vi "Initialize Drive System.vi"(6 "RightDriveMaster":u8, 7 "LeftDriveMaster":u8, 8 "RightDriveSlave1":u8, 9 "RightDriveSlave2":u8, 10 "LeftDriveSlave 2":u8, 11 "LeftDriveSlave1":u8) -> (1 "RightDriveMaster":T1, 2 "LeftDriveMaster":T1)   [LabVIEW 2018]
uses:
  <vilib>/Rock Robotics/WPI/MotorControl/WPI_MotorControlDeviceRef.ctl
  <vilib>/Rock Robotics/WPI/MotorControl/WPI_MotorControlType.ctl
  <vilib>/Rock Robotics/SystemInterfaces/DIO/FPGA_DIOPWMChannel.ctl
  <vilib>/Rock Robotics/WPI/PWM/WPI_PWMDeadband.ctl
  <vilib>/Rock Robotics/SystemInterfaces/DIO/FPGA_DIOChannel.ctl
  <vilib>/Rock Robotics/WPI/ThirdParty/Phoenix-LabVIEW/Motor Controller/Controls/CTRE_Phoenix_MotorControl_NeutralMode.ctl
  Infrastructure/Constants.vi
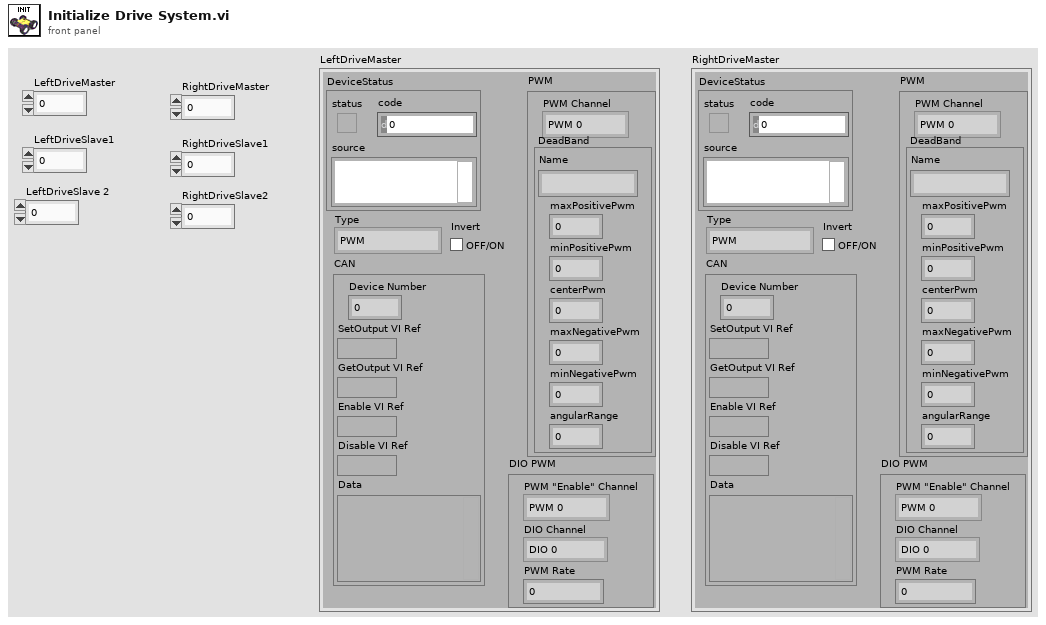
[diagram p1: front panel]
types:
  T1 = typedef "WPI_MotorControlDeviceRef.ctl" = cluster{"DeviceStatus":errorcluster, "Type":T2, "PWM":cluster{"PWM Channel":T3, "DeadBand":T4}, "CAN":cluster{"Device Number":u8, "SetOutput VI Ref":variant, "GetOutput VI Ref":variant, "Enable VI Ref":variant, "Disable VI Ref":variant, "Data":variant}, "Invert":bool, "DIO PWM":cluster{"PWM \"Enable\" Channel":T3, "DIOChannel":T5, "PWM Rate":dbl}}
  T2 = typedef "WPI_MotorControlType.ctl" = enum16{"PWM", "CAN", "DIO PWM"}
  T3 = typedef "FPGA_DIOPWMChannel.ctl" = enum8{"PWM 0", "PWM 1", "PWM 2", "PWM 3", "PWM 4", "PWM 5", "PWM 6", "PWM 7", "PWM 8", "PWM 9", "PWM MXP 0", "PWM MXP 1", "PWM MXP 2", "PWM MXP 3", "PWM MXP 4", "PWM MXP 5", "PWM MXP 6", "PWM MXP 7", "PWM MXP 8", "PWM MXP 9", "Invalid"}
  T4 = typedef "WPI_PWMDeadband.ctl" = cluster{"Name":string, "maxPositivePwm":i32, "minPositivePwm":i32, "centerPwm":i32, "maxNegativePwm":i32, "minNegativePwm":i32, "angularRange":u16}
  T5 = typedef "FPGA_DIOChannel.ctl" = enum8{"DIO 0", "DIO 1", "DIO 2", "DIO 3", "DIO 4", "DIO 5", "DIO 6", "DIO 7", "DIO 8", "DIO 9", "DIO MXP 0", "DIO MXP 1", "DIO MXP 2", "DIO MXP 3", "DIO MXP 4", "DIO MXP 5", "DIO MXP 6", "DIO MXP 7", "DIO MXP 8", "DIO MXP 9", "DIO MXP 10", "DIO MXP 11", "DIO MXP 12", "DIO MXP 13", "DIO MXP 14", "DIO MXP 15", "SPI Port CS1", "SPI Port CS2", "SPI Port CS3", "SPI Port MISO", "SPI Port MOSI", "Invalid"}
  T6 = typedef "CTRE_Phoenix_MotorControl_NeutralMode.ctl" = enum8{"EEPROMSetting", "Override to Coast", "Override to Brake"}
  T7 = enum16{"FollowerType_PercentOutput", "FollowerType_AuxOutput1"}
  T8 = cluster{"Cruise Velocity":i32, "Acceleration":i32}
  T9 = cluster{"P":dbl, "I":dbl, "D":dbl, "F":dbl, "I Zone":dbl}
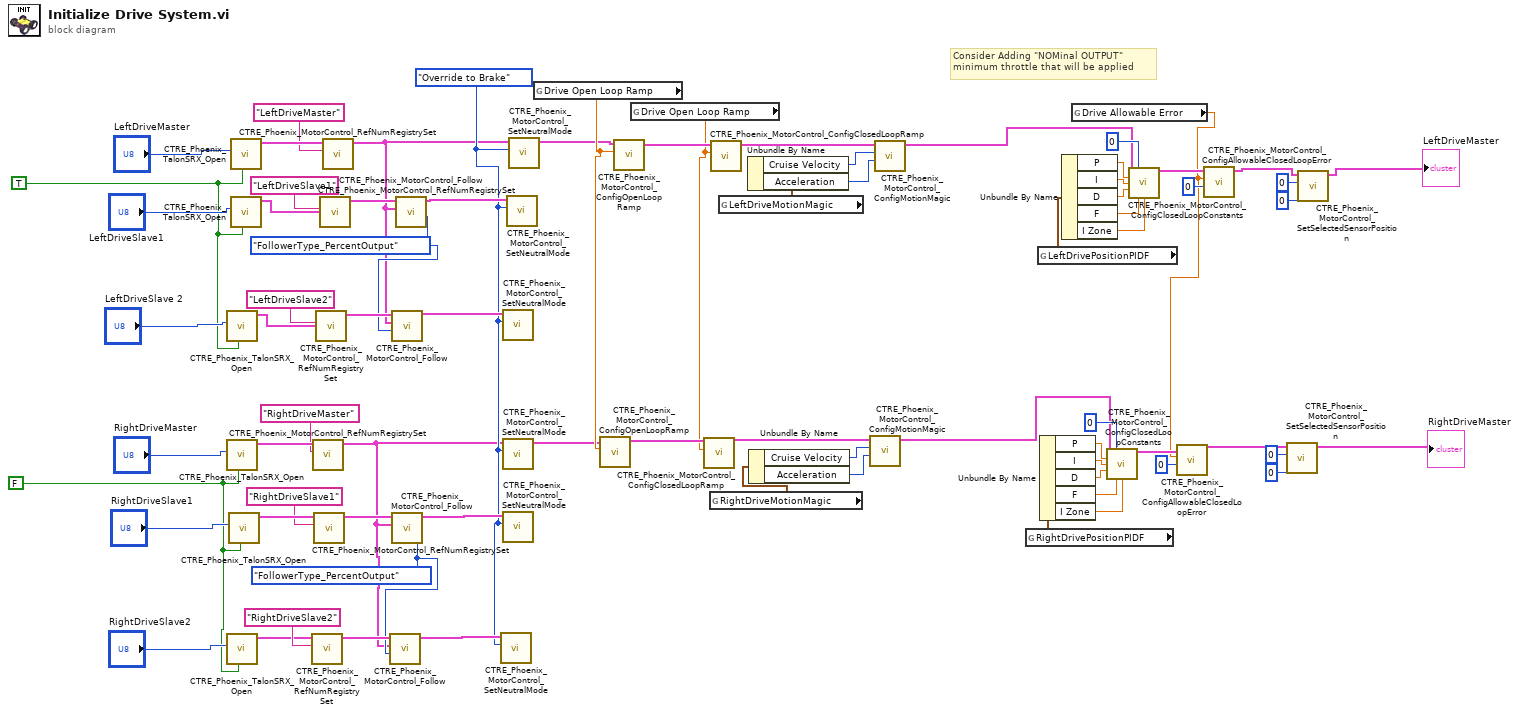
[diagram p0: block diagram]
diagram:
  w27 = FALSE
  w28 = TRUE
  w31 = CTRE_Phoenix_MotorControl_NeutralMode."Override to Brake" ("Motor Control Neutral Mode")
  w33 = T7."FollowerType_PercentOutput" ("FollowerType")
  w32 = T7."FollowerType_PercentOutput" ("FollowerType")
  # "Consider Adding \"NOMinal OUTPUT\" \nminimum throttle that will be applied"
  n1 = call <vilib>:"CTRE_Phoenix_TalonSRX_Open.vi"("Invert"=w28, "Device Number"="LeftDriveSlave 2") -> ("CAN Talon SRX Ref"=w39:T1)  [unwired: 8 in, 1 out]
  n2 = call <vilib>:"CTRE_Phoenix_TalonSRX_Open.vi"("Invert"=w27, "Device Number"="RightDriveMaster") -> ("CAN Talon SRX Ref"=w52:T1)  [unwired: 8 in, 1 out]
  n3 = call <vilib>:"CTRE_Phoenix_TalonSRX_Open.vi"("Invert"=w27, "Device Number"="RightDriveSlave2") -> ("CAN Talon SRX Ref"=w34:T1)  [unwired: 8 in, 1 out]
  n4 = call <vilib>:"CTRE_Phoenix_TalonSRX_Open.vi"("Invert"=w27, "Device Number"="RightDriveSlave1") -> ("CAN Talon SRX Ref"=w57:T1)  [unwired: 8 in, 1 out]
  n5 = call <vilib>:"CTRE_Phoenix_TalonSRX_Open.vi"("Invert"=w28, "Device Number"="LeftDriveMaster") -> ("CAN Talon SRX Ref"=w53:T1)  [unwired: 8 in, 1 out]
  n6 = call <vilib>:"CTRE_Phoenix_TalonSRX_Open.vi"("Invert"=w28, "Device Number"="LeftDriveSlave1") -> ("CAN Talon SRX Ref"=w59:T1)  [unwired: 8 in, 1 out]
  n7 = call <vilib>:"CTRE_Phoenix_MotorControl_RefNumRegistrySet.vi"("refnum name"="RightDriveSlave2", "PhoenixMotorControlDevRef"=w34) -> ("PhoenixMotorControlDevRef"=w37:T1)  [unwired: 8 in, 1 out]
  n8 = call <vilib>:"CTRE_Phoenix_MotorControl_RefNumRegistrySet.vi"("refnum name"="RightDriveMaster", "PhoenixMotorControlDevRef"=w52) -> ("PhoenixMotorControlDevRef"=w29:T1)  [unwired: 8 in, 1 out]
  n9 = call <vilib>:"CTRE_Phoenix_MotorControl_RefNumRegistrySet.vi"("refnum name"="RightDriveSlave1", "PhoenixMotorControlDevRef"=w57) -> ("PhoenixMotorControlDevRef"=w46:T1)  [unwired: 8 in, 1 out]
  n10 = call <vilib>:"CTRE_Phoenix_MotorControl_RefNumRegistrySet.vi"("refnum name"="LeftDriveSlave2", "PhoenixMotorControlDevRef"=w39) -> ("PhoenixMotorControlDevRef"=w42:T1)  [unwired: 8 in, 1 out]
  n11 = call <vilib>:"CTRE_Phoenix_MotorControl_RefNumRegistrySet.vi"("refnum name"="LeftDriveSlave1", "PhoenixMotorControlDevRef"=w59) -> ("PhoenixMotorControlDevRef"=w47:T1)  [unwired: 8 in, 1 out]
  n12 = call <vilib>:"CTRE_Phoenix_MotorControl_RefNumRegistrySet.vi"("refnum name"="LeftDriveMaster", "PhoenixMotorControlDevRef"=w53) -> ("PhoenixMotorControlDevRef"=w30:T1)  [unwired: 8 in, 1 out]
  n13 = call <vilib>:"CTRE_Phoenix_MotorControl_Follow.vi"("FollowerType"=w33, "Master Controller to Follow"=w29, "PhoenixMotorControlDevRef"=w37) -> ("PhoenixMotorControlDevRef"=w38:T1)  [unwired: 7 in, 1 out]
  n14 = call <vilib>:"CTRE_Phoenix_MotorControl_Follow.vi"("FollowerType"=w32, "Master Controller to Follow"=w30, "PhoenixMotorControlDevRef"=w42) -> ("PhoenixMotorControlDevRef"=w43:T1)  [unwired: 7 in, 1 out]
  n15 = call <vilib>:"CTRE_Phoenix_MotorControl_Follow.vi"("FollowerType"=w33, "Master Controller to Follow"=w29, "PhoenixMotorControlDevRef"=w46) -> ("PhoenixMotorControlDevRef"=w45:T1)  [unwired: 7 in, 1 out]
  n16 = call <vilib>:"CTRE_Phoenix_MotorControl_Follow.vi"("FollowerType"=w32, "Master Controller to Follow"=w30, "PhoenixMotorControlDevRef"=w47) -> ("PhoenixMotorControlDevRef"=w44:T1)  [unwired: 7 in, 1 out]
  n17 = call <vilib>:"CTRE_Phoenix_MotorControl_SetNeutralMode.vi"("Motor Control Neutral Mode"=w31, "PhoenixMotorControlDevRef"=w38) -> ()  [unwired: 8 in, 2 out]
  n18 = call <vilib>:"CTRE_Phoenix_MotorControl_SetNeutralMode.vi"("Motor Control Neutral Mode"=w31, "PhoenixMotorControlDevRef"=w43) -> ()  [unwired: 8 in, 2 out]
  n19 = call <vilib>:"CTRE_Phoenix_MotorControl_SetNeutralMode.vi"("Motor Control Neutral Mode"=w31, "PhoenixMotorControlDevRef"=w29) -> ("PhoenixMotorControlDevRef"=w60:T1)  [unwired: 8 in, 1 out]
  n20 = call <vilib>:"CTRE_Phoenix_MotorControl_SetNeutralMode.vi"("Motor Control Neutral Mode"=w31, "PhoenixMotorControlDevRef"=w45) -> ()  [unwired: 8 in, 2 out]
  n21 = call <vilib>:"CTRE_Phoenix_MotorControl_SetNeutralMode.vi"("Motor Control Neutral Mode"=w31, "PhoenixMotorControlDevRef"=w44) -> ()  [unwired: 8 in, 2 out]
  n22 = call <vilib>:"CTRE_Phoenix_MotorControl_SetNeutralMode.vi"("Motor Control Neutral Mode"=w31, "PhoenixMotorControlDevRef"=w30) -> ("PhoenixMotorControlDevRef"=w61:T1)  [unwired: 8 in, 1 out]
  n23 = global read "Constants.vi" "Drive Open Loop Ramp"() -> (w62:dbl)
  n24 = call <vilib>:"CTRE_Phoenix_MotorControl_ConfigOpenLoopRamp.vi"("secondsFromNeutralToFull"=w62, "PhoenixMotorControlDevRef"=w60) -> ("PhoenixMotorControlDevRef"=w24:T1)  [unwired: 8 in, 1 out]
  n25 = call <vilib>:"CTRE_Phoenix_MotorControl_ConfigOpenLoopRamp.vi"("secondsFromNeutralToFull"=w62, "PhoenixMotorControlDevRef"=w61) -> ("PhoenixMotorControlDevRef"=w26:T1)  [unwired: 8 in, 1 out]
  n26 = global read "Constants.vi" "Drive Open Loop Ramp"() -> (w22:dbl)
  n27 = call <vilib>:"CTRE_Phoenix_MotorControl_ConfigClosedLoopRamp.vi"("secondsFromNeutralToFull"=w22, "PhoenixMotorControlDevRef"=w24) -> ("PhoenixMotorControlDevRef"=w23:T1)  [unwired: 8 in, 1 out]
  n28 = global read "Constants.vi" "RightDriveMotionMagic"() -> (w18:T8)
  n29 = call <vilib>:"CTRE_Phoenix_MotorControl_ConfigClosedLoopRamp.vi"("secondsFromNeutralToFull"=w22, "PhoenixMotorControlDevRef"=w26) -> ("PhoenixMotorControlDevRef"=w25:T1)  [unwired: 8 in, 1 out]
  n30 = global read "Constants.vi" "LeftDriveMotionMagic"() -> (w21:T8)
  n31 = Unbundle By Name(w21) -> ("Cruise Velocity"=w20:i32, "Acceleration"=w19:i32)
  n32 = Unbundle By Name(w18) -> ("Cruise Velocity"=w17:i32, "Acceleration"=w16:i32)
  n33 = call <vilib>:"CTRE_Phoenix_MotorControl_ConfigMotionMagic.vi"("Acceleration"=w16, "Cruise Velocity"=w17, "PhoenixMotorControlDevRef"=w23) -> ("PhoenixMotorControlDevRef"=w15:T1)  [unwired: 7 in, 1 out]
  n34 = call <vilib>:"CTRE_Phoenix_MotorControl_ConfigMotionMagic.vi"("Acceleration"=w19, "Cruise Velocity"=w20, "PhoenixMotorControlDevRef"=w25) -> ("PhoenixMotorControlDevRef"=w14:T1)  [unwired: 7 in, 1 out]
  n35 = global read "Constants.vi" "RightDrivePositionPIDF"() -> (w73:T9)
  n36 = global read "Constants.vi" "LeftDrivePositionPIDF"() -> (w63:T9)
  n37 = Unbundle By Name(w73) -> ("P"=w72:dbl, "I"=w71:dbl, "D"=w74:dbl, "F"=w75:dbl, "I Zone"=w76:dbl)
  n38 = Unbundle By Name(w63) -> ("P"=w64:dbl, "I"=w65:dbl, "D"=w66:dbl, "F"=w67:dbl, "I Zone"=w68:dbl)
  n39 = global read "Constants.vi" "Drive Allowable Error"() -> (w9:dbl)
  n40 = call <vilib>:"CTRE_Phoenix_MotorControl_ConfigClosedLoopConstants.vi"("PhoenixMotorControlDevRef"=w15, "slotIdx"=0, "P"=w72, "I"=w71, "D"=w74, "F"=w75, "I Zone"=w76) -> ("PhoenixMotorControlDevRef"=w12:T1)  [unwired: 7 in, 1 out]
  n41 = call <vilib>:"CTRE_Phoenix_MotorControl_ConfigClosedLoopConstants.vi"("PhoenixMotorControlDevRef"=w14, "slotIdx"=0, "P"=w64, "I"=w65, "D"=w66, "F"=w67, "I Zone"=w68) -> ("PhoenixMotorControlDevRef"=w13:T1)  [unwired: 7 in, 1 out]
  n42 = call <vilib>:"CTRE_Phoenix_MotorControl_ConfigAllowableClosedLoopError.vi"("slotIdx"=u32 0, "allowableClosedLoopError"=w9, "PhoenixMotorControlDevRef"=w12) -> ("PhoenixMotorControlDevRef"=w8:T1)  [unwired: 7 in, 1 out]
  n43 = call <vilib>:"CTRE_Phoenix_MotorControl_ConfigAllowableClosedLoopError.vi"("slotIdx"=u32 0, "allowableClosedLoopError"=w9, "PhoenixMotorControlDevRef"=w13) -> ("PhoenixMotorControlDevRef"=w3:T1)  [unwired: 7 in, 1 out]
  n44 = call <vilib>:"CTRE_Phoenix_MotorControl_SetSelectedSensorPosition.vi"("pidLoopIdx"=u32 0, "New Sensor Position"=0, "PhoenixMotorControlDevRef"=w8) -> ("PhoenixMotorControlDevRef"=→"RightDriveMaster":T1)  [unwired: 7 in, 1 out]
  n45 = call <vilib>:"CTRE_Phoenix_MotorControl_SetSelectedSensorPosition.vi"("pidLoopIdx"=u32 0, "New Sensor Position"=0, "PhoenixMotorControlDevRef"=w3) -> ("PhoenixMotorControlDevRef"=→"LeftDriveMaster":T1)  [unwired: 7 in, 1 out]
